vi "getSignalOut.vi"(6 "Delay between send and receive [ms]":i32=100, 8 "error in (no error)":errorcluster, 11 "CCD in":refnum<class "CCD.lvclass">) -> (0 "error out":errorcluster, 1 "signalType":i32, 2 "event":i32, 3 "CCD out":refnum<class "CCD.lvclass">, 5 "address":i32)   [LabVIEW 2023, in "CCD.lvclass"]
doc: "ccd_getSignalOut\nThis command is used to get the current setting of the signal output. The address, event, and signalType parameters are used to define the signal based on the supported options of that particular CCD.\nThe supported signal options are retrieved using the ccd_getConfig command, and begin with the \"Signals\" string contained in the configuration.\nFor example:\n\n\"signals\": [\n {\n \"events\": [\n {\n \"name\": \"Shutter Open\",\n \"token\": 3,\n \"types\": [\n {\n \"name\": \"TTL Active Low\",\n \"token\": 1\n },\n {\n \"name\": \"TTL Active High\",\n \"token\": 0\n }\n ]\n },\n {\n \"name\": \"Start Experiment\",\n \"token\": 0,\n \"types\": [\n {\n \"name\": \"TTL Active Low\",\n \"token\": 1\n },\n {\n \"name\": \"TTL Active High\",\n \"token\": 0\n }\n ]\n }\n ],\n \"name\": \"Signal Output\",\n \"token\": 0\n }\n]"
uses:
  CCD.lvclass
  SignalOut.ctl
  20f7d3bd-08ac-4524-9bed-df36c1da25a0.vi
  a21955fc-e3a0-4e36-8495-41f1bfac7860.vi
  <vilib>/JDP Science/JSONtext/Variant to JSON Text.vi
  <vilib>/JDP Science/JSONtext/Set Item.vi
  <vilib>/JDP Science/JSONtext/JSON text to Variant.vi
  <vilib>/JDP Science/JSONtext/LVClass Serializer/JSONtext LVClass Serializer.lvclass
  CCD.lvclass/CCD.ctl
  GenericDevice/GenericDevice.lvclass
panel:
  # "Connector Pane"
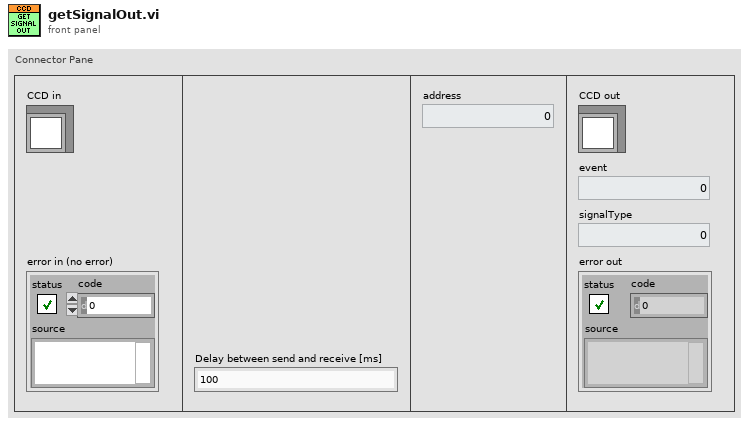
[diagram p1: front panel]
types:
  T1 = typedef "CCD.lvclass/SignalOut.ctl" = cluster{"address":i32, "event":i32, "signalType":i32}
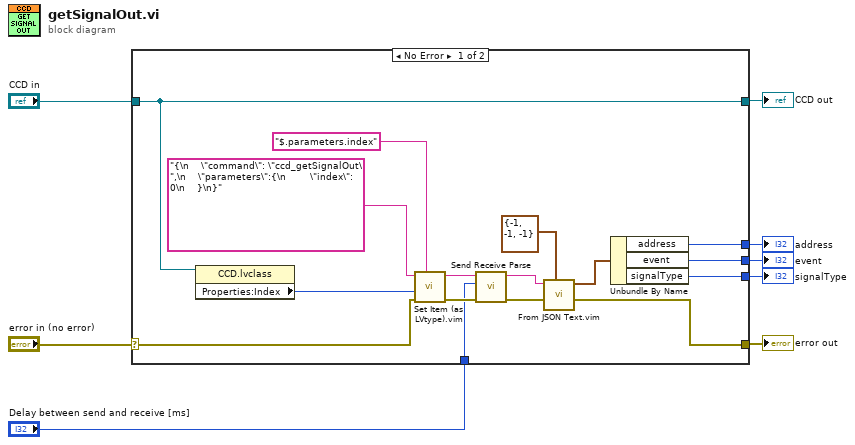
[diagram p0: block diagram]
diagram:
  n1 = case shown="No Error" "error in (no error)" {
    selector: "error in (no error)" -> [w20 w26]
    tunnel: [w19 w26] -> w7
    tunnel: [w22 w25] -> w5
    tunnel: "CCD in" -> [w22 w25]
    tunnel: "Delay between send and receive [ms]" -> [w13 _]
    tunnel: [w11 _] -> w3
    tunnel: [w10 _] -> w2
    tunnel: [w9 _] -> w1
    frame No Error {
      n2 = property class="CCD.lvclass"(reference=w22) -> ("Properties:Index"=w21:i32)  [unwired: 1 in, 2 out]
      n3 = call "Set Item (as LVtype).vim"("$Path or Item Name"="$.parameters.index", "error in (no error)"=w20, "Anything"=w21, "JSON"="{\n    \"command\": \"ccd_getSignalOut\",\n    \"parameters\":{\n        \"index\": 0\n    }\n}") -> ("error out"=w16:errorcluster, "<JSON>"=w18:string)  [unwired: 4 in, 1 out]
      n4 = call "Send Receive Parse.vi"("error in"=w16, "Delay between send and receive [ms]"=w13, "<JSON>"=w18) -> ("error out"=w15:errorcluster, "results-JSON string"=w17:string)  [unwired: 6 in, 1 out]
      n5 = call "From JSON Text.vim"("Data Type and Default Value"=T1 {"address"=-1, "event"=-1, "signalType"=-1} ("Trigger Parameters"), "error in (no error)"=w15, "JSON"=w17) -> ("error out"=w19:errorcluster, "Data out"=w14:T1)  [unwired: 7 in]
      n6 = Unbundle By Name(w14) -> ("address"=w10:i32, "event"=w11:i32, "signalType"=w9:i32)
    }
    frame Error {
    }
  }
  "error out" <- w7
  "CCD out" <- w5
  "event" <- w3
  "address" <- w2
  "signalType" <- w1
